vi "Is Calling VI Running.vi"(8 "Error In":errorcluster, 11 "Calling VI Name":string) -> (0 "Error Out":errorcluster, 3 "Running?":bool)   [LabVIEW 2019, in "Notebook.lvlib"]
uses:
  Notebook.lvlib
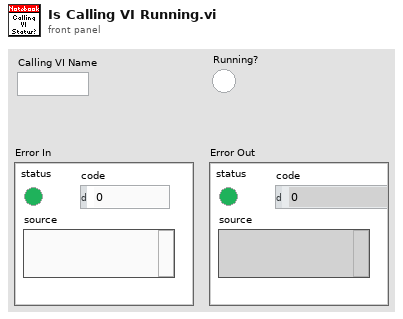
[diagram p1: front panel]
types:
  T1 = enum32{"Bad", "Idle", "Run top level", "Running"}[]
  T2 = enum32{"Bad", "Idle", "Run top level", "Running"}
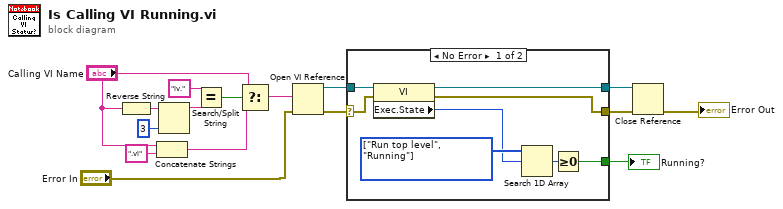
[diagram p0: block diagram]
diagram:
  n1 = Reverse String(1:"Calling VI Name") -> (0:w16:string)
  n2 = Concatenate Strings("Calling VI Name", ".vi" ("string")) -> (w9:string)
  n3 = Search/Split String(string=w16, offset (0)=3) -> (substring before match=w14:string)  [unwired: 1 in, 2 out]
  n4 = Equal?(x="iv.", y=w14) -> (x = y?=w12:bool)
  n5 = Select(t="Calling VI Name", s=w12, f=w9) -> (s? t:f=w2:string)
  n6 = Open VI Reference(vi path=w2, error in (no error)="Error In") -> (vi reference=w8:refnum<vi>, error out=w6:errorcluster)  [unwired: 4 in]
  n7 = case shown="No Error" w6 {
    selector: w6 -> [w22 w25]
    tunnel: w8 -> [w24 w26]
    tunnel: [w23 w26] -> w7
    tunnel: [w17 _] -> w5
    tunnel: [w21 w25] -> w4
    frame No Error {
      w20 = T1 [enum."Run top level", enum."Running"] items=["Bad", "Idle", "Run top level", "Running"] ("Execution:State")
      n8 = property class="VI"(reference=w24, error in=w22) -> (reference out=w23:refnum<vi>, error out=w21:errorcluster, "Exec.State"=w19:T2)
      n9 = Search 1D Array(1D array=w20, element=w19) -> (index of element=w18:i32)  [unwired: 1 in]
      n10 = Greater Or Equal To 0?(x=w18) -> (x >= 0?=w17:bool)
    }
    frame Error {
    }
  }
  "Running?" <- w5
  n11 = Close Reference(reference=w7, error in (no error)=w4) -> (error out=→"Error Out":errorcluster)
